vi "Table_flush.vi"(4 "唯一元素列索引":dbl, 5 "唯一列元素？":bool, 8 "输入数据":string[](array[string]), 9 "表格引用":refnum<vi>) -> (0 "修正重复？":bool)   [LabVIEW 2019]
panel:
  # "选T:数据对应列不会有重复，有重复输入是更新历史项\n  F:普通的增加数据到历史数据，增加新一行"
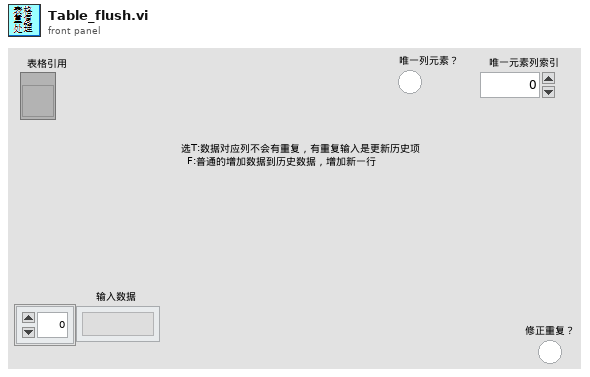
[diagram p1: front panel]
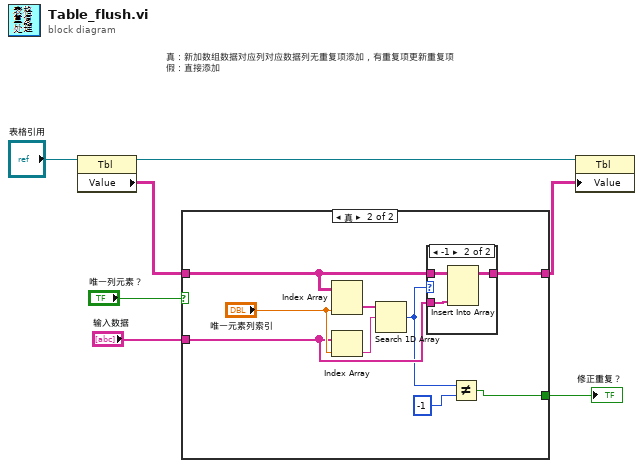
[diagram p0: block diagram]
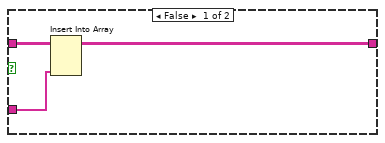
[diagram p2: hidden frame]
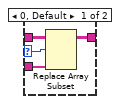
[diagram p3: hidden frame]
diagram:
  # "真：新加数组数据对应列对应数据列无重复项添加，有重复项更新重复项\n假：直接添加"
  n1 = property class="Tbl"(reference="表格引用") -> (reference out=w2:refnum<vi>, "Value"=w5:string[][])  [unwired: 1 in, 1 out]
  n2 = case shown="真" "唯一列元素？" {
    tunnel: w5 -> [w10 w16]
    tunnel: [w8 w15] -> w4
    tunnel: "输入数据" -> [w9 w14]
    tunnel: [_ w11] -> w1
    frame False {
      n3 = Insert Into Array(array=w10, new element=w9) -> (w8:string[][])  [unwired: 2 in]
    }
    frame True {
      n4 = Index Array(array=w16, index (col)="唯一元素列索引") -> (element=w18:string[])  [unwired: 1 in]
      n5 = Index Array(array=w14, index="唯一元素列索引") -> (element=w17:string)
      n6 = Search 1D Array(1D array=w18, element=w17) -> (index of element=w13:i32)  [unwired: 1 in]
      n7 = case shown="-1" w13 {
        selector: w13 -> [w23 _]
        tunnel: w16 -> [w22 w26]
        tunnel: w14 -> [w21 w25]
        tunnel: [w20 w24] -> w15
        frame 0, Default {
          n8 = Replace Array Subset(array=w22, new element=w21, index (row)=w23) -> (w20:string[][])  [unwired: 1 in]
        }
        frame -1 {
          n9 = Insert Into Array(array=w26, new element=w25) -> (w24:string[][])  [unwired: 2 in]
        }
      }
      n10 = Not Equal?(x=w13, y=-1) -> (x != y?=w11:bool)
    }
  }
  "修正重复？" <- w1
  n11 = property class="Tbl"(reference=w2, "Value"=w4) -> ()  [unwired: 1 in, 2 out]
